vi "encoder.vi"   [LabVIEW 2015]
uses:
  <vilib>/Erdos Miller/LV-JSON/Parse JSON String (JSON).vi
  src/lib/TOML.lvlib
  <vilib>/Erdos Miller/LV-JSON/LV-JSON.lvlib
types:
  T1 = typedef "LV-JSON.lvlib/JSON Value.ctl" = cluster{"\\type":enum16{"Object", "Array", "String", "Number", "Boolean", "Null"}, "ÿýÿýÿýÿýÿýÿþÿýÿýÿý&LV-JSON.lvlib:JSON Name-Value Pair.ctlÿýÿýÿýÿýÿýÿþÿýÿýÿýLV-JSON.lvlib:JSON Value.ctl":variant}
  T2 = typedef "TOML.lvlib/TOML Value.ctl" = cluster{"\\type":enum16{"Table", "Array", "String", "Integer", "Float", "Boolean", "Offset Date-Time", "Local Date-Time", "Local Date", "Local Time"}, "ÿýÿýÿýÿýÿýÿþÿýÿýÿý%LV-TOML.lvlib:TOML Key-Value Pair.ctlÿýÿýÿýÿýÿýÿþÿýÿýÿýLV-TOML.lvlib:TOML Value.ctl$":variant}
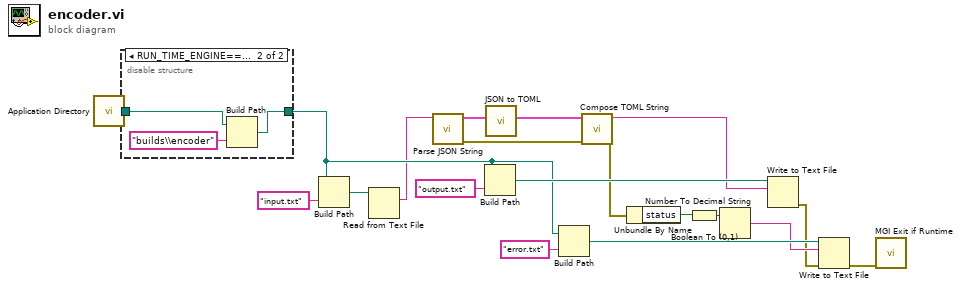
[diagram p0: block diagram]
diagram:
  n1 = call <vilib>:"Application Directory.vi"() -> ("Application Directory"=w16:path)
  n2 = disable-structure shown="RUN_TIME_ENGINE==False" {
    disable-tunnel: [w20 w22] -> w11
    disable-tunnel: w16 -> [w20 w23]
    frame condition #0 {
    }
    frame condition #1 (active) {
      n3 = Build Path(base path=w23, name or relative path="builds\\encoder") -> (appended path=w22:path)
    }
  }
  n4 = Build Path(base path=w11, name or relative path="input.txt") -> (appended path=w18:path)
  n5 = Read from Text File(file (use dialog)=w18) -> (text=w6:string)  [unwired: 3 in, 3 out]
  n6 = call-poly <vilib>:"Parse JSON String.vi"("String"=w6) -> ("error out"=w2:errorcluster, "Value"=w4:T1)  [unwired: 9 in]
  n7 = Build Path(base path=w11, name or relative path="output.txt") -> (appended path=w14:path)
  n8 = call "JSON to TOML.vi"("JSON Value"=w4) -> ("Value"=w3:T2)  [unwired: 10 in]
  n9 = Build Path(base path=w11, name or relative path="error.txt") -> (appended path=w12:path)
  n10 = call "Compose TOML String.vi"("error in (no error)"=w2, "Value"=w3) -> ("error out"=w1:errorcluster, "String"=w5:string)  [unwired: 8 in]
  n11 = Unbundle By Name(w1) -> ("status"=w13:bool)
  n12 = Boolean To (0,1)(Boolean=w13) -> (0, 1=w7:i16)
  n13 = Number To Decimal String(number=w7) -> (decimal integer string=w10:string)  [unwired: 1 in]
  n14 = Write to Text File(file (use dialog)=w14, text=w5) -> (error out=w9:errorcluster)  [unwired: 2 in, 2 out]
  n15 = Write to Text File(file (use dialog)=w12, text=w10, error in=w9) -> (error out=w8:errorcluster)  [unwired: 1 in, 2 out]
  n16 = call <userlib>:"MGI Exit if Runtime.vi"("Error In (Dependency Only)"=w8) -> ()  [unwired: 11 in]
